vi "State Memory Operation.vi"(8 "error in (no error)":errorcluster, 9 "Register (0: Register 0)":u16(ring) items=["Register 0", "Register 1", "Register 2", "Register 3", "Register 4", "Register 5", "Register 6", "Register 7", "Register 8", "Register 9", "Register 10", "Register 11", "Register 12", "Register 13", "Register 14", "Register 15", "Register 16", "Register 17", "Register 18", "Register 19"], 10 "Operation (0: Store)":u16(ring) items=["Store", "Load", "Delete"], 11 "VISA resource name":refnum<visa-resource-name>) -> (0 "error out":errorcluster, 3 "VISA resource name out":refnum<visa-resource-name>)   [LabVIEW 2016, in "Agilent E4980.lvlib"]
doc: "The memory operations based on the specified register number include:\n\n(1) Stores the configuration state to the memories.\n(2) Loads the configuration state to the memories.\n(3) Deletes the configuration state from the memories."
uses:
  <instrlib>/Agilent E4980/Agilent E4980.lvlib
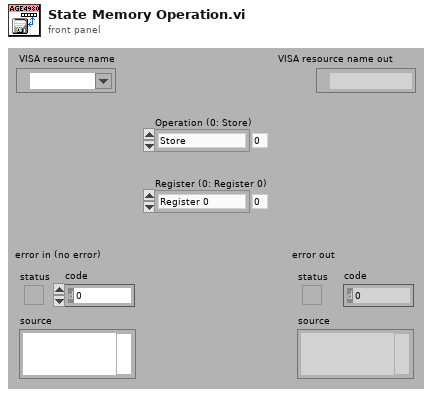
[diagram p1: front panel]
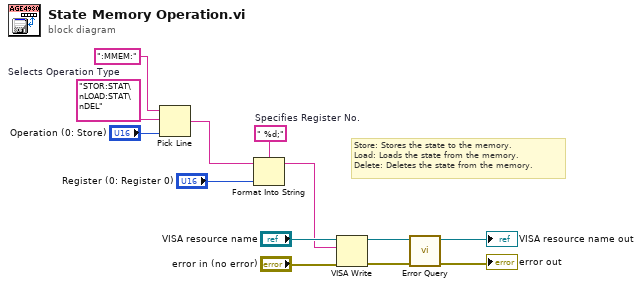
[diagram p0: block diagram]
diagram:
  w11 = " %d;"  # Specifies Register No.
  w1 = "STOR:STAT\nLOAD:STAT\nDEL"  # Selects Operation Type
  # "Store: Stores the state to the memory.\nLoad: Loads the state from the memory.\nDelete: Deletes the state from the memory."
  n1 = Pick Line(string ("")=":MMEM:", multi-line string=w1, line index="Operation (0: Store)") -> (output string=w9:string)
  n2 = Format Into String(format string=w11, initial string=w9, "Register (0: Register 0)") -> (resulting string=w6:string)  [unwired: 1 in, 1 out]
  n3 = VISA Write(VISA resource name="VISA resource name", write buffer=w6, error in (no error)="error in (no error)") -> (VISA resource name out=w5:refnum<visa-resource-name>, error out=w4:errorcluster)  [unwired: 1 out]
  n4 = call <instrlib>:"Error Query.vi"("error in (no error)"=w4, "VISA resource name"=w5) -> ("error out"=→"error out":errorcluster, "VISA resource name out"=→"VISA resource name out":refnum<visa-resource-name>)  [unwired: 6 in, 2 out]
